vi "SubVI_Img2MatGrey_001.vi"(0 "Path":path) -> (1 "Picture":picture, 2 "1-bit pixmap":bool[][](array[boolean]))   [LabVIEW 2018]
panel:
  out "mask":u8[](array[numeric])
  out "24-bit pixmap":u32[][](array[numeric]) format="%x"
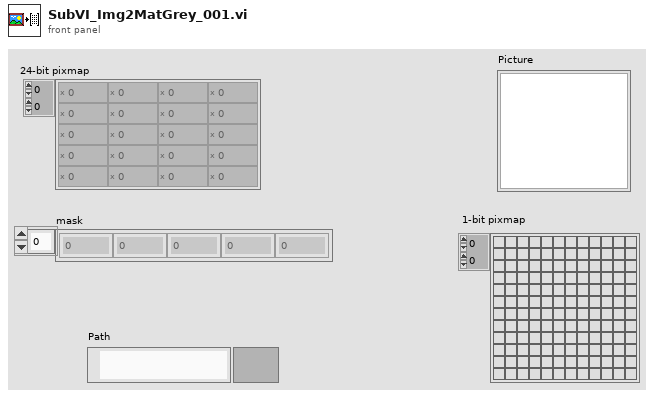
[diagram p1: front panel]
types:
  T1 = typedef "imagedata.ctl" = cluster{"image type":i32, "image depth":i32, "image":u8[], "mask":u8[], "colors":u32[], "Rectangle":cluster{"left":i16, "top":i16, "right":i16, "bottom":i16}}
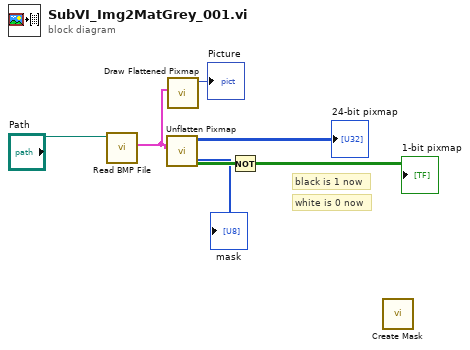
[diagram p0: block diagram]
diagram:
  # "white is 0 now"
  # "black is 1 now"
  n1 = call <vilib>:"Read BMP File.vi"("path to BMP file"="Path") -> ("image data"=w4:T1)  [unwired: 8 in, 2 out]
  n2 = call <vilib>:"Unflatten Pixmap.vi"("image data"=w4) -> ("1-bit pixmap"=w6:bool[][], "24-bit pixmap"=→"24-bit pixmap":u32[][], "mask"=→"mask":u8[])  [unwired: 4 in, 4 out]
  n3 = call <vilib>:"Draw Flattened Pixmap.vi"("image data"=w4) -> ("new picture"=→"Picture":picture)  [unwired: 8 in]
  n4 = Not(x=w6) -> (.not. x?=→"1-bit pixmap":bool[][])
  n5 = call <vilib>:"Create Mask.vi"() -> ()  [unwired: 11 in, 1 out]
